vi "CPU_DDC.vi"(5 "anti-aliasing?":bool=TRUE, 6 "FIR filter specifications":T1={"alias rejection (dB)"=120.0, "normalized bandwidth"=0.2}, 7 "reset":bool, 8 "error in (no error)":errorcluster, 9 "resample factor":cluster{"interpolation":i32, "decimation":i32}={"interpolation"=1, "decimation"=50}, 10 "Freq Offset":sgl=21320.0, 11 "Array":cdb[](array[numeric])) -> (0 "error out":errorcluster, 3 "Y":cdb[](array[numeric]))   [LabVIEW 2020]
uses:
  <vilib>/Analysis/2dsp.llb/Rational Resample (single channel, CDB).vi
  <vilib>/Analysis/NI_AALPro.lvlib
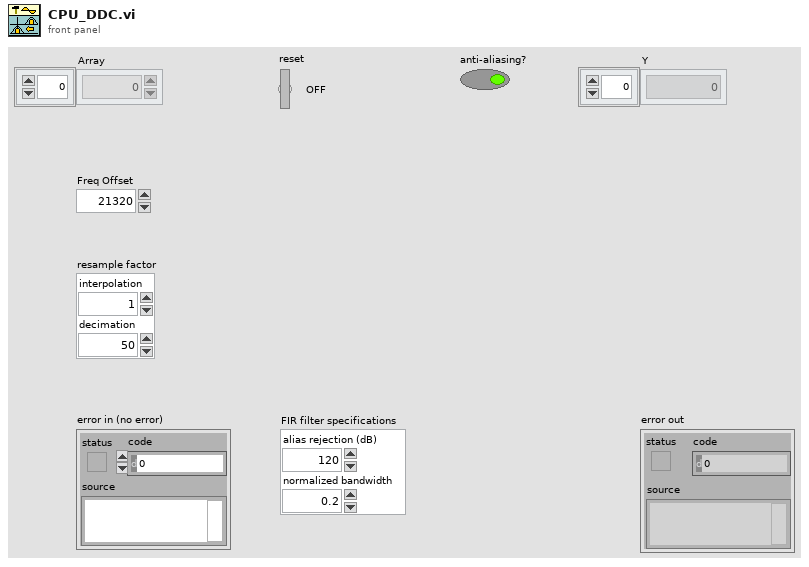
[diagram p1: front panel]
types:
  T1 = cluster{"alias rejection (dB)":dbl, "normalized bandwidth":dbl}
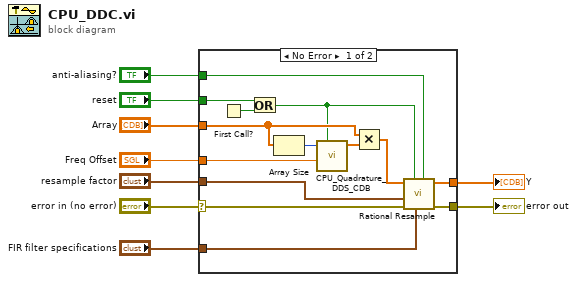
[diagram p0: block diagram]
diagram:
  n1 = case shown="No Error" "error in (no error)" {
    selector: "error in (no error)" -> [w15 w24]
    tunnel: "resample factor" -> [w23 _]
    tunnel: "FIR filter specifications" -> [w22 _]
    tunnel: "Array" -> [w21 _]
    tunnel: [w20 _] -> w6
    tunnel: "anti-aliasing?" -> [w16 _]
    tunnel: "reset" -> [w12 _]
    tunnel: [w14 w24] -> w2
    tunnel: "Freq Offset" -> [w13 _]
    frame No Error {
      n2 = First Call?() -> (First Call?: T/F=w10:bool)
      n3 = Or(x=w12, y=w10) -> (x .or. y?=w11:bool)
      n4 = Array Size(array=w21) -> (size(s)=w19:i32)
      n5 = call "CPU_Quadrature_DDS_CDB.vi"("reset"=w11, "Freq Offset"=w13, "size"=w19) -> ("T1D_CSG out"=w18:cdb[])  [unwired: 7 in, 1 out]
      n6 = Multiply(x=w21, y=w18) -> (x*y=w17:cdb[])
      n7 = call-poly <vilib>:"Rational Resample.vi"("anti-aliasing?"=w16, "FIR filter specifications"=w22, "reset"=w11, "error in (no error)"=w15, "resample factor"=w23, "X"=w17) -> ("error out"=w14:errorcluster, "Y"=w20:cdb[])  [unwired: 3 in, 1 out]
    }
    frame Error {
    }
  }
  "Y" <- w6
  "error out" <- w2
